vi "Voice Recorder.vi"() -> ()   [LabVIEW 2015]
uses:
  <vilib>/sound2/lvsound2.llb/Sound Data Format.ctl
  <vilib>/sound2/lvsound2.llb/Sound File Write Open.vi
  <vilib>/sound2/lvsound2.llb/Sound File Write (DBL Single).vi
  <vilib>/Analysis/NI_AAL_SigProc.lvlib
panel:
  out "Numeric":dbl
  out "LowPass Filtered Voice":dynamicdata(graph)
  out "Original Raw Voice":dynamicdata(graph)
  in  "Sound Format":T1={"sample rate (S/s)"=22050.0, "number of channels"=2, "bits per sample"=16}
  out "Numeric 2":dbl
  in  "peaks/valleys":enum32{"Peaks", "Valleys"}(ring)
  in  "stop":bool
  # "Voice Recorder"
  # "by Anni Blair, Edith Acosta, Kris Bickham"
  # "Original Raw Voice"
  # "LowPass Filtered Voice"
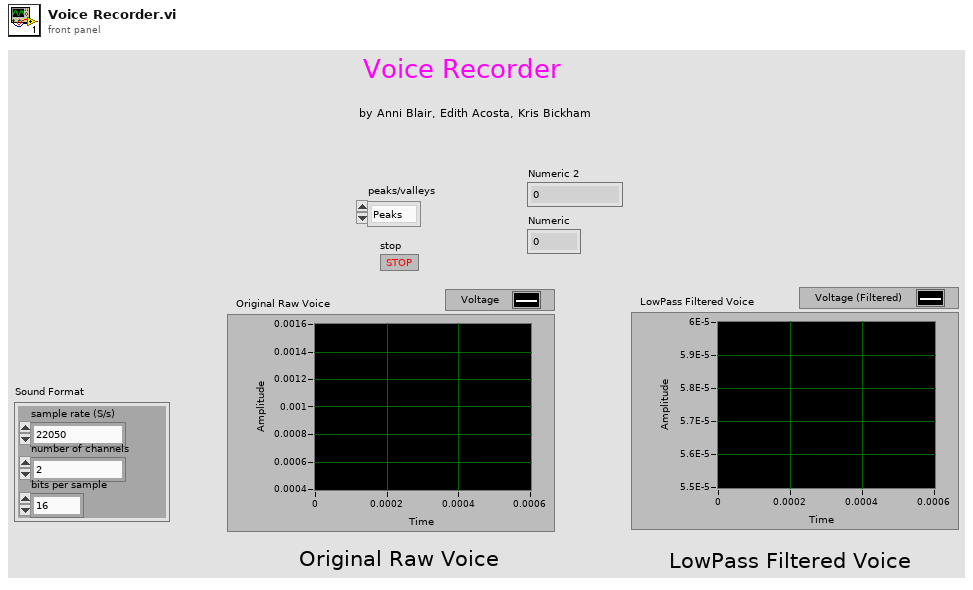
[diagram p1: front panel]
types:
  T1 = typedef "Sound Data Format.ctl" = cluster{"sample rate (S/s)":dbl, "number of channels":i32, "bits per sample":i32}
  T2 = typedef "Sound File Refnum.ctl" = refnum<file>
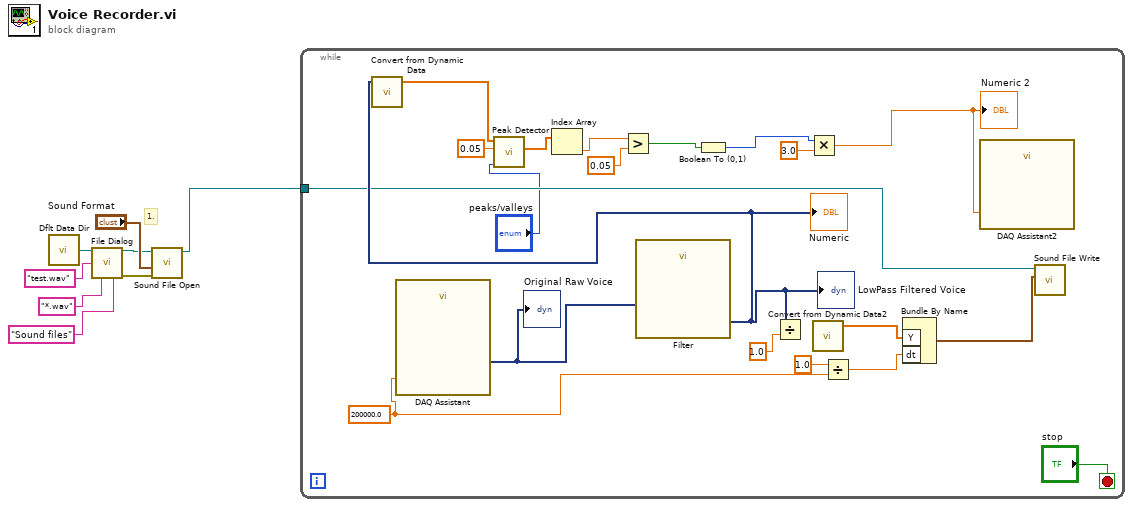
[diagram p0: block diagram]
diagram:
  # "1."
  n1 = call <vilib>:"Dflt Data Dir.vi"() -> ("App:Default Data Directory"=w7:path)
  n2 = call "File Dialog"("start path"=w7, "default name"="test.wav", "pattern (all files)"="*.wav" ("DNL_pattern"), "pattern label"="Sound files") -> ("selected path"=w4:path, "error out"=w3:errorcluster)  [unwired: 8 in, 2 out]
  n3 = call-poly <vilib>:"Sound File Open.vi"("error in (no error)"=w3, "sound format"="Sound Format", "path"=w4) -> ("sound file refnum"=w1:T2)  [unwired: 7 in, 1 out]
  n4 = while {
    tunnel: w1 -> [w13]
    stop <- "stop" stop-if-true
    w11 = 200000.0 ("y")
    n5 = call "DAQ Assistant"("rate"=w11) -> ("data"=w10:dynamicdata)  [unwired: 15 in, 3 out]
    "Original Raw Voice" <- w10
    n6 = call "Filter"("Signal"=w10) -> ("Filtered Signal"=w14:dynamicdata)  [unwired: 9 in, 1 out]
    "LowPass Filtered Voice" <- w14
    "Numeric" <- w14
    n7 = call "Convert from Dynamic Data"("Dynamic Data Type"=w14) -> ("Array"=w19:dbl[])  [unwired: 3 in]
    n8 = call <vilib>:"Peak Detector.vi"("peaks/valleys"="peaks/valleys", "threshold"=0.05, "X"=w19) -> ("Amplitudes"=w26:dbl[])  [unwired: 4 in, 4 out]
    n9 = Index Array(array=w26) -> (element=w25:dbl)  [unwired: 1 in]
    n10 = Greater?(x=w25, y=0.05) -> (0:w23:bool)
    n11 = Boolean To (0,1)(Boolean=w23) -> (0, 1=w21:i16)
    n12 = Divide(x=w14, y=1.0) -> ()  [unwired: 1 out]
    n13 = Multiply(x=w21, y=3.0) -> (x*y=w9:dbl)
    "Numeric 2" <- w9
    n14 = call "Convert from Dynamic Data2"() -> ("Array"=w18:dbl[])  [unwired: 4 in]
    n15 = Divide(x=1.0, y=w11) -> (x/y=w17:dbl)
    n16 = Bundle By Name("Y"=w18, "dt"=w17) -> (w20:waveform(dbl))  [unwired: 1 in]
    n17 = call "DAQ Assistant2"("data"=w9) -> ()  [unwired: 17 in, 2 out]
    n18 = call-poly <vilib>:"Sound File Write.vi"("data"=w20, "sound file refnum"=w13) -> ()  [unwired: 8 in, 2 out]
  }
